vi "E10_Manejo de string.vi"() -> ()   [LabVIEW 2026]
panel:
  out "after substring 2":string
  out "offset past match":dbl
  out "after substring":string
  out "match substring":string
  out "before substring":string
  out "result string 1":string
  out "result string 2":string
  out "result":string
  out "String":string
  out "Numeric":dbl
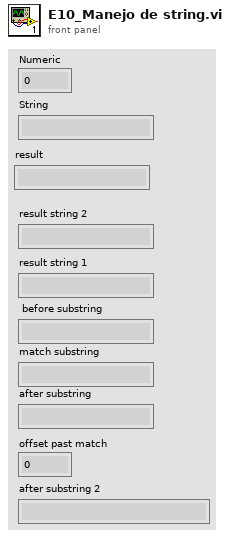
[diagram p1: front panel]
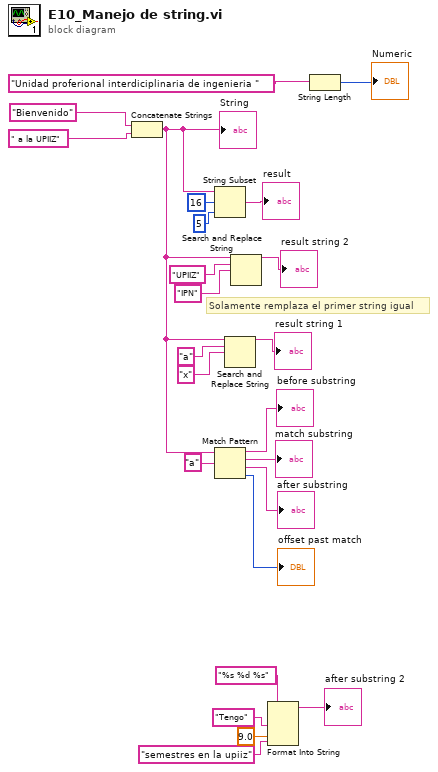
[diagram p0: block diagram]
diagram:
  # "Solamente remplaza el primer string igual"
  n1 = Concatenate Strings("Bienvenido" ("String"), " a la UPIIZ" ("String")) -> (w7:string)
  "String" <- w7
  n2 = String Subset(string=w7, offset (0)=16, length (rest)=5 ("offset (0)")) -> (substring=→"result":string)
  n3 = Match Pattern(string=w7, regular expression="a" ("String")) -> (before substring=→"before substring":string, match substring=→"match substring":string, after substring=→"after substring":string, offset past match=→"offset past match":i32)  [unwired: 1 in]
  n4 = Search and Replace String(input string=w7, search string="a" ("String"), replace string="x" ("String")) -> (result string=→"result string 1":string)  [unwired: 5 in, 3 out]
  n5 = Search and Replace String(input string=w7, search string="UPIIZ" ("String"), replace string="IPN" ("String")) -> (result string=→"result string 2":string)  [unwired: 5 in, 3 out]
  n6 = Format Into String(format string="%s %d %s" ("String"), "Tengo" ("String"), 9.0 ("input 1"), "semestres en la upiiz" ("String")) -> (resulting string=→"after substring 2":string)  [unwired: 2 in, 1 out]
  n7 = String Length(string="Unidad proferional interdiciplinaria de ingenieria " ("String")) -> (length=→"Numeric":i32)
